vi "update.vi"(8 "error in (no error)":errorcluster, 11 "Context in":refnum<class "Context.lvclass">) -> (0 "error out":errorcluster, 3 "Context out":refnum<class "Context.lvclass">)   [LabVIEW 2013, in "Context.lvclass"]
uses:
  Context.lvclass
  Context.lvclass/Context.ctl
  State/State.lvclass
  Model/Model/Model.lvclass
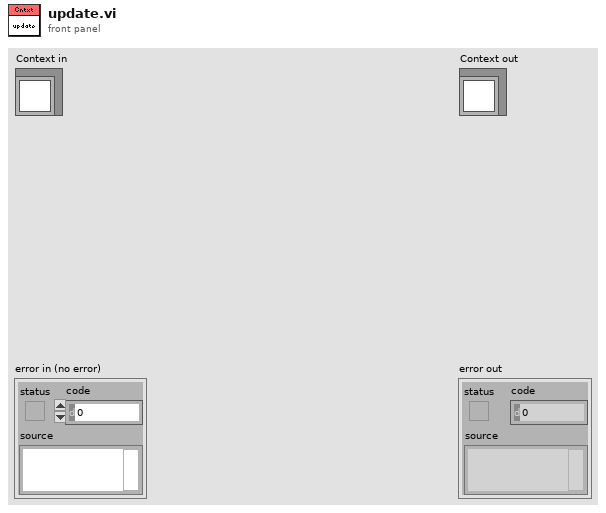
[diagram p1: front panel]
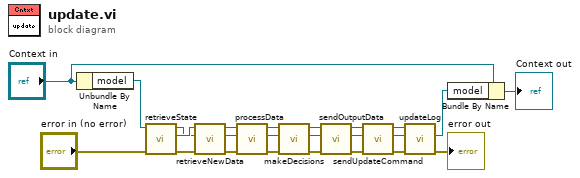
[diagram p0: block diagram]
diagram:
  n1 = Unbundle By Name("Context in") -> ("model"=w24:refnum<class "Model.lvclass">)
  n2 = call "retrieveState.vi"("error in (no error)"="error in (no error)", "Model in"=w24) -> ("error out"=w16:errorcluster, "state"=w20:refnum<class "State.lvclass">, "Model out"=w18:refnum<class "Model.lvclass">)  [unwired: 7 in]
  n3 = call-dynamic "retrieveNewData.vi"("error in (no error)"=w16, "model"=w18, "State in"=w20) -> ("error out"=w15:errorcluster, "model 2"=w17:refnum<class "Model.lvclass">, "State out"=w19:refnum<class "State.lvclass">)  [unwired: 6 in]
  n4 = call-dynamic "processData.vi"("error in (no error)"=w15, "model"=w17, "State in"=w19) -> ("error out"=w6:errorcluster, "model 2"=w5:refnum<class "Model.lvclass">, "State out"=w4:refnum<class "State.lvclass">)  [unwired: 6 in]
  n5 = call-dynamic "makeDecisions.vi"("error in (no error)"=w6, "model"=w5, "State in"=w4) -> ("error out"=w1:errorcluster, "model 2"=w2:refnum<class "Model.lvclass">, "State out"=w3:refnum<class "State.lvclass">)  [unwired: 6 in]
  n6 = call-dynamic "sendOutputData.vi"("error in (no error)"=w1, "model"=w2, "State in"=w3) -> ("error out"=w8:errorcluster, "model 2"=w7:refnum<class "Model.lvclass">, "State out"=w9:refnum<class "State.lvclass">)  [unwired: 6 in]
  n7 = call-dynamic "sendUpdateCommand.vi"("error in (no error)"=w8, "model"=w7, "State in"=w9) -> ("error out"=w12:errorcluster, "model 2"=w13:refnum<class "Model.lvclass">, "State out"=w14:refnum<class "State.lvclass">)  [unwired: 6 in]
  n8 = call-dynamic "updateLog.vi"("error in (no error)"=w12, "model"=w13, "State in"=w14) -> ("error out"=→"error out":errorcluster, "model 2"=w10:refnum<class "Model.lvclass">)  [unwired: 6 in, 1 out]
  n9 = Bundle By Name(cluster="Context in", "model"=w10) -> (→"Context out":refnum<class "Context.lvclass">)
